vi "CNT Material Properties.vi"(6 "m-nm CNT":dbl, 9 "CNT Thickness (CNT Length)":dbl, 10 "Energy (Heat; I^2R)":dbl, 11 "NS Base Area":dbl) -> (1 "Mass CNTs":dbl, 2 "Delta Temp Change CNT":dbl, 3 "CNT Specfic Heat Capacity":dbl, 4 "CNT Density":dbl, 5 "Volume CNT":dbl, 7 "CNT Thickness":dbl)   [LabVIEW 2020]
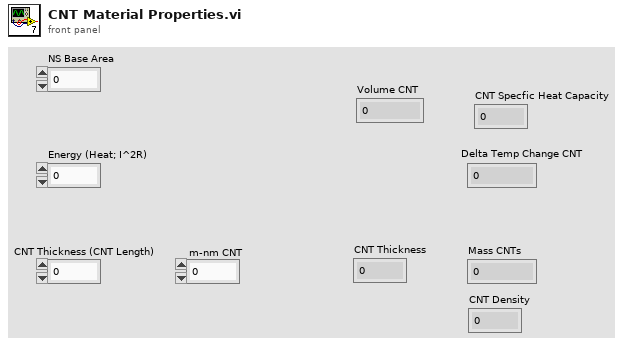
[diagram p1: front panel]
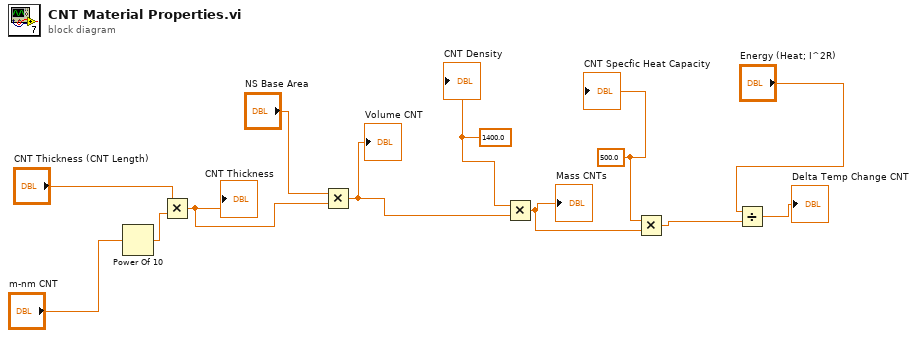
[diagram p0: block diagram]
diagram:
  w12 = 500.0 ("Silicon Specfic Heat Capacity 7")
  w5 = 1400.0 ("Silicon Density 7")
  n1 = Power Of 10(x="m-nm CNT") -> (10^x=w1:dbl)
  n2 = Multiply(x="CNT Thickness (CNT Length)", y=w1) -> (x*y=w4:dbl)
  "CNT Thickness" <- w4
  n3 = Multiply(x="NS Base Area", y=w4) -> (x*y=w6:dbl)
  "Volume CNT" <- w6
  n4 = Multiply(x=w5, y=w6) -> (x*y=w11:dbl)
  "Mass CNTs" <- w11
  n5 = Multiply(x=w12, y=w11) -> (x*y=w10:dbl)
  n6 = Divide(x="Energy (Heat; I^2R)", y=w10) -> (x/y=→"Delta Temp Change CNT":dbl)
  "CNT Density" <- w5
  "CNT Specfic Heat Capacity" <- w12
